vi "Wedge.vi"(8 "error in":errorcluster) -> (0 "error out":errorcluster)   [LabVIEW 2015]
uses:
  Sprocket/src/Refname/Queues.ctl
  Sprocket/src/Refname/Actuators.ctl
  Sprocket/src/Action/Action Name.ctl
  Sprocket/src/Refname/Refname to String (Queue).vi
  Sprocket/lib/Sprocket.lvlib
panel:
  in  "Wedge steady":dbl=-0.05
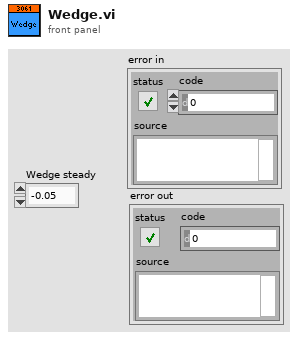
[diagram p1: front panel]
types:
  T1 = typedef "Sprocket.lvlib/Actuators.ctl" = enum16{"Drive Motor 1 (R)", "Drive Motor 2 (R)", "Drive Motor 3 (R)", "Drive Motor 4 (L)", "Drive Motor 5 (L)", "Drive Motor 6 (L)", "Collector Motor", "Collector Solenoid", "Compressor", "SonicShifter", "Gyro", "UltraSonic Front Left", "UltraSonic Back Left", "Wedge Motor", "Wedge LS"}
  T2 = typedef "Sprocket.lvlib/Queues.ctl" = enum16{"Input", "Drive", "Collector", "Shifter", "Wedge"}
  T3 = typedef "WPI_SwitchDevRef.ctl" = cluster{"DevStatus":errorcluster, "DIO Channel":T4, "CntIndex":T5, "Normally Closed":bool}
  T4 = typedef "FPGA_DIOChannel.ctl" = enum8{"DIO 0", "DIO 1", "DIO 2", "DIO 3", "DIO 4", "DIO 5", "DIO 6", "DIO 7", "DIO 8", "DIO 9", "DIO MXP 0", "DIO MXP 1", "DIO MXP 2", "DIO MXP 3", "DIO MXP 4", "DIO MXP 5", "DIO MXP 6", "DIO MXP 7", "DIO MXP 8", "DIO MXP 9", "DIO MXP 10", "DIO MXP 11", "DIO MXP 12", "DIO MXP 13", "DIO MXP 14", "DIO MXP 15", "Invalid"}
  T5 = typedef "FPGA_CounterCtrSystemIndex.ctl" = enum8{"Ctr 0", "Ctr 1", "Ctr 2", "Ctr 3", "Ctr 4", "Ctr 5", "Ctr 6", "Ctr 7", "Invalid"}
  T6 = typedef "WPI_MotorControlDeviceRef.ctl" = cluster{"DeviceStatus":errorcluster, "Type":T7, "PWM":cluster{"PWM Channel":T8, "DeadBand":T9}, "CAN":cluster{"Device Number":u8, "Control Mode":T10, "Semaphore":T11, "Max Vout":dbl, "TalonSRX Control Mode":T12}, "Invert":bool}
  T7 = typedef "WPI_MotorControlType.ctl" = enum16{"PWM", "CAN", "CANTalonSRX"}
  T8 = typedef "FPGA_DIOPWMChannel.ctl" = enum8{"PWM 0", "PWM 1", "PWM 2", "PWM 3", "PWM 4", "PWM 5", "PWM 6", "PWM 7", "PWM 8", "PWM 9", "PWM MXP 0", "PWM MXP 1", "PWM MXP 2", "PWM MXP 3", "PWM MXP 4", "PWM MXP 5", "PWM MXP 6", "PWM MXP 7", "PWM MXP 8", "PWM MXP 9", "Invalid"}
  T9 = typedef "WPI_PWMDeadband.ctl" = cluster{"Name":string, "maxPositivePwm":i32, "minPositivePwm":i32, "centerPwm":i32, "maxNegativePwm":i32, "minNegativePwm":i32, "angularRange":u16}
  T10 = typedef "WPI_CANJaguar_ControlMode.ctl" = enum8{"Percent VBus", "Current", "Speed", "Position", "Voltage"}
  T11 = typedef "Semaphore RefNum" = refnum<k1>
  T12 = typedef "WPI_CANTalonSRX_APIControlMode.ctl" = enum8{"Percent VBus", "Speed", "Position", "Slave", "Unchanged / Invalid", "Voltage Compensation", "Current", "Motion Profile"}
  T13 = typedef "Sprocket.lvlib/Action Name.ctl" = enum16{"No Action", "Drive Train Both", "Drive Train Rotate", "Drive Train Throttle", "Collector Motor Roll", "Collector Motor Eject", "Collector Motor Collect", "Collector Motor Stop", "Collector Extend", "Collector Retract", "Shifter High", "Shifter Low", "Collector Motor Stall", "Wedge Roll"}
  T14 = typedef "Sprocket.lvlib/Action.ctl" = cluster{"Name":T13, "Priority":i32, "Data":variant}
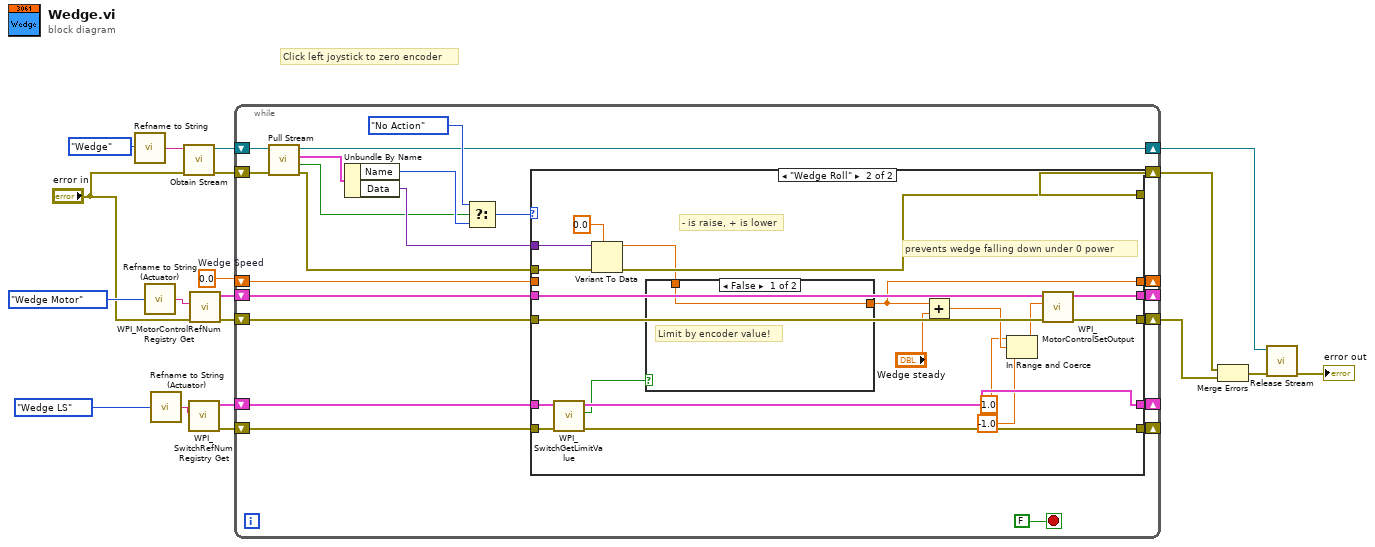
[diagram p0: block diagram]
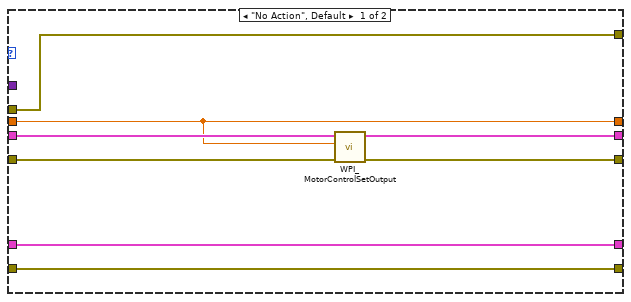
[diagram p2: hidden frame]
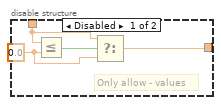
[diagram p4: hidden frame]
diagram:
  w8 = 0.0  # Wedge Speed
  # "Click left joystick to zero encoder"
  n1 = call-poly "Refname to String.vi"("Queue Refname"=Queues."Wedge" ("Refname (Queue)")) -> ("Refnum Name"=w18:string)
  n2 = call "Refname to String (Actuator).vi"("Actuator Refname"=Actuators."Wedge Motor") -> ("Refnum Name"=w12:string)
  n3 = call "Refname to String (Actuator).vi"("Actuator Refname"=Actuators."Wedge LS") -> ("Refnum Name"=w3:string)
  n4 = call "Obtain Stream.vi"("error in (no error)"="error in", "Name"=w18) -> ("error out"=w16:errorcluster, "stream out"=w17:refnum<queue>)  [unwired: 8 in]
  n5 = call <vilib>:"WPI_SwitchRefNum Registry Get.vi"("refnum name"=w3) -> ("error out"=w1:errorcluster, "SwitchDevRef"=w2:T3)  [unwired: 9 in]
  n6 = call <vilib>:"WPI_MotorControlRefNum Registry Get.vi"("error in (no error)"="error in", "refnum name"=w12) -> ("error out"=w10:errorcluster, "MotorControlDevRef"=w11:T6)  [unwired: 8 in]
  n7 = while {
    shift-right: [w36] -> w14
    shift-left: w17 -> [w41]
    shift-right: [w29] -> _
    shift-left: w11 -> [w30]
    shift-right: [w28] -> w5
    shift-left: w10 -> [w31]
    shift-right: [w27] -> w6
    shift-left: w16 -> [w40]
    shift-right: [w26] -> _
    shift-left: w8 -> [w25]
    shift-right: [w22] -> _
    shift-left: w2 -> [w24]
    shift-right: [w21] -> _
    shift-left: w1 -> [w23]
    stop <- FALSE stop-if-true
    n8 = call "Pull Stream.vi"("error in (no error)"=w40, "stream in"=w41) -> ("error out"=w32:errorcluster, "timed out?"=w20:bool, "element"=w37:T14, "queue out"=w36:refnum<queue>)  [unwired: 6 in]
    n9 = Unbundle By Name(w37) -> ("Name"=w39:T13, "Data"=w33:variant)
    n10 = Select(t=Action_Name."No Action" ("Name"), s=w20, f=w39) -> (s? t:f=w34:T13)
    n11 = case shown="\"Wedge Roll\"" w34 {
      tunnel: w33 -> [_ w69]
      tunnel: w32 -> [w49 w63]
      tunnel: w31 -> [w47 w66]
      tunnel: w30 -> [w48 w67]
      tunnel: [w46 w65] -> w29
      tunnel: [w45 w64] -> w28
      tunnel: [w49 w62] -> w27
      tunnel: [w44 w55] -> w26
      tunnel: w25 -> [w44 _]
      tunnel: w24 -> [w43 w61]
      tunnel: w23 -> [w42 w60]
      tunnel: [w43 w59] -> w22
      tunnel: [w42 w58] -> w21
      frame "No Action", Default {
        n12 = call <vilib>:"WPI_MotorControlSetOutput.vi"("error in (no error)"=w47, "Output"=w44, "MotorControlDevRef"=w48) -> ("error out"=w45:errorcluster, "MotorControlDevRef"=w46:T6)  [unwired: 6 in, 1 out]
      }
      frame "Wedge Roll" {
        # "prevents wedge falling down under 0 power"
        # "- is raise, + is lower"
        n13 = call <vilib>:"WPI_SwitchGetLimitValue.vi"("error in (no error)"=w60, "SwitchDevRef"=w61) -> ("error out"=w58:errorcluster, "Switch Pressed"=w57:bool, "SwitchDevRef"=w59:T3)  [unwired: 7 in]
        n14 = Variant To Data(error in=w63, type=0.0, Variant=w69) -> (data=w56:dbl, error out=w62:errorcluster)
        n15 = case shown="False" w57 {
          tunnel: w56 -> [w70 w72]
          tunnel: [w70 w71] -> w55
          frame False {
            # "Limit by encoder value!"
          }
          frame True {
            n16 = disable-structure shown="Enabled" {
              disable-tunnel: w72 -> [w75 w77]
              disable-tunnel: [w73 w77] -> w71
              frame Disabled {
                w74 = 0.0 ("y")
                # "Only allow - values"
                n17 = Less Or Equal?(x=w75, y=w74) -> (x <= y?=w76:bool)
                n18 = Select(t=w75, s=w76, f=w74) -> (s? t:f=w73:dbl)
              }
              frame Enabled {
              }
            }
          }
        }
        n19 = Add(x=w55, y="Wedge steady") -> (x+y=w53:dbl)
        n20 = In Range and Coerce(upper limit=1.0, x=w53, lower limit=-1.0) -> (coerced(x)=w50:dbl)  [unwired: 1 out]
        n21 = call <vilib>:"WPI_MotorControlSetOutput.vi"("error in (no error)"=w66, "Output"=w50, "MotorControlDevRef"=w67) -> ("error out"=w64:errorcluster, "MotorControlDevRef"=w65:T6)  [unwired: 6 in, 1 out]
      }
    }
  }
  n22 = Merge Errors(w6, w5) -> (w7:errorcluster)
  n23 = call "Release Stream.vi"("error in (no error)"=w7, "stream in"=w14) -> ("error out"=→"error out":errorcluster)  [unwired: 8 in, 1 out]
